vi "VCI Read Err Info.vi"(8 "error in (no error)":errorcluster, 9 "CANIndex":u32, 10 "DevIndex":u32, 11 "DevType":u32) -> (0 "error out":errorcluster, 2 "function return":u32, 3 "pErrInfo":T1)   [LabVIEW 2012, in "ControlCAN.lvlib"]
doc: "unsigned int WINAPI VCI_ReadErrInfo(unsigned int DevType,unsigned int DevIndex,unsigned int CANIndex,PVCI_ERR_INFO pErrInfo);"
uses:
  ControlCAN.lvlib
  Ginkgo_Driver.dll
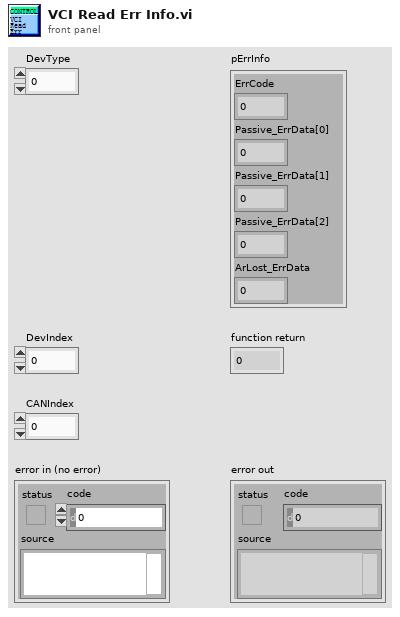
[diagram p1: front panel]
types:
  T1 = cluster{"ErrCode":u32, "Passive_ErrData[0]":u8, "Passive_ErrData[1]":u8, "Passive_ErrData[2]":u8, "ArLost_ErrData":u8}
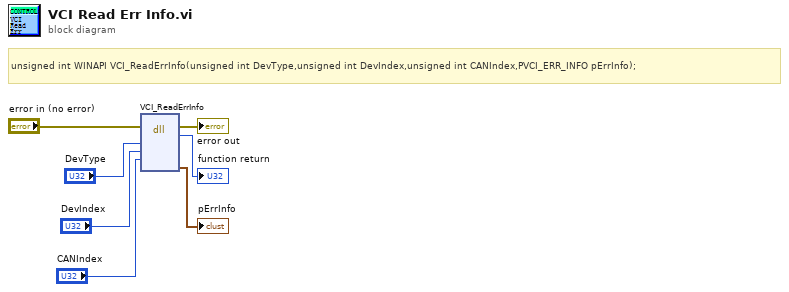
[diagram p0: block diagram]
diagram:
  # "unsigned int WINAPI VCI_ReadErrInfo(unsigned int DevType,unsigned int DevIndex,unsigned int CANIndex,PVCI_ERR_INFO pErrInfo);"
  n1 = dll-call lib="E:/Project/vt_ginkgo/truck/Ginkgo Driver/vs2010/Ginkgo_USB-I2C_API_v2.0.3.0/lib/labview_64bit/ControlCAN/Ginkgo_Driver.*" fn="VCI_ReadErrInfo"(error in="error in (no error)", "DevType"="DevType", "DevIndex"="DevIndex", "CANIndex"="CANIndex") -> (error out=→"error out":errorcluster, →"function return":u32, "pErrInfo"=→"pErrInfo":T1)  [unwired: 6 in, 1 out]
